vi "Event handler-Motor Z button.vi"(11 "Motor Z button's value":bool) -> (0 "error out":errorcluster)   [LabVIEW 2020]
uses:
  Typedefs/Top level VI states.ctl
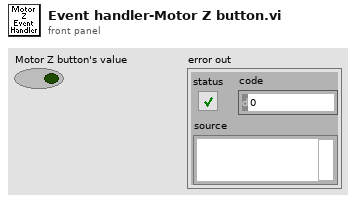
[diagram p1: front panel]
types:
  T1 = typedef "Top level VI states.ctl" = enum16{"None", "Initialise UI", "<STACK PROTOCOL STATES>", "AOL Zstack-START", "AOL Zstack-STOP", "Motor Zstack-START", "Motor Zstack-STOP", "<ACQUISITION PROTOCOL STATES> ", "Functional Acquisition-START", "Functional Acquisition-STOP", "Single Plane Acquisition-START", "Single Plane Acquisition-STOP", "Volume Acquisition-START", "Volume Acquisition-STOP", "<LIVE IMAGING PROTOCOL STATES>", "Live Imaging-START", "Live Imaging-STOP", "Live Plane Imaging-START", "Live Plane Imaging-STOP", "Live Volume Imaging-START", "Live Volume Imaging-STOP", "<MOVEMENT CORRECTION PROTOCOL STATES>", "EXIT"}
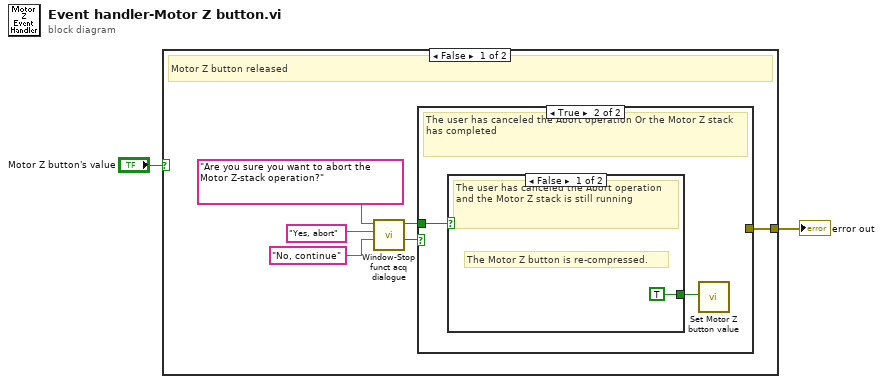
[diagram p0: block diagram]
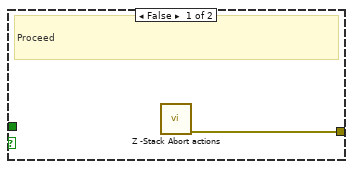
[diagram p2: hidden frame]
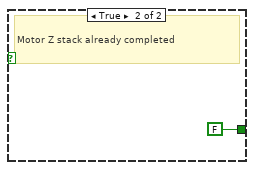
[diagram p3: hidden frame]
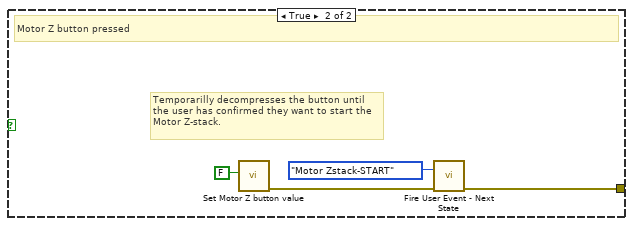
[diagram p4: hidden frame]
diagram:
  n1 = case shown="False" "Motor Z button's value" {
    tunnel: [w3 w15] -> w1
    frame False {
      # "Motor Z button released"
      n2 = call "Window-Stop funct acq dialogue.vi"("Caption-Left button (Cancel)"="No, continue", "Caption-Right button (OK)"="Yes, abort", "Message string"="Are you sure you want to abort the Motor Z-stack operation?") -> ("User canceled the Abort Or the func acqcompleted"=w8:bool, "Funct acq completed"=w4:bool)  [unwired: 6 in, 1 out]
      n3 = case shown="True" w8 {
        tunnel: [w9 _] -> w3
        tunnel: w4 -> [_ w11]
        frame False {
          # "Proceed"
          n4 = call "Z -Stack Abort actions.vi"() -> ("error out"=w9:errorcluster)  [unwired: 11 in]
        }
        frame True {
          # "The user has canceled the Abort operation Or the Motor Z stack has completed"
          n5 = case shown="False" w11 {
            tunnel: [TRUE ("Value") FALSE ("Value")] -> w10
            frame False {
              # "The Motor Z button is re-compressed."
              # "The user has canceled the Abort operation and the Motor Z stack is still running"
            }
            frame True {
              # "Motor Z stack already completed"
            }
          }
          n6 = call "Set Motor Z button value.vi"("Motor Z button's new value"=w10) -> ()  [unwired: 10 in, 1 out]
        }
      }
    }
    frame True {
      # "Temporarilly decompresses the button until the user has confirmed they want to start the Motor Z-stack."
      # "Motor Z button pressed"
      n7 = call "Set Motor Z button value.vi"("Motor Z button's new value"=FALSE ("Value")) -> ("error out"=w14:errorcluster)  [unwired: 10 in]
      n8 = call "Fire User Event - Next State.vi"("Error In"=w14, "\"UI Handler loop\" case to execute"=Top_level_VI_states."Motor Zstack-START" ("event data / imaging mode")) -> ("Error Out"=w15:errorcluster)  [unwired: 9 in]
    }
  }
  "error out" <- w1
